vi "Byte Buffer.Read (1D I64).vi"(8 "error in (no error)":errorcluster, 9 "count":i32, 10 "buffer offset":i32, 11 "Byte Buffer in":refnum<class "Byte Buffer.lvclass">) -> (0 "error out":errorcluster, 1 "value":i64[](array[numeric]), 3 "Byte Buffer out":refnum<class "Byte Buffer.lvclass">)   [LabVIEW 2016, in "VeriStand Data.lvlib" / "Byte Buffer.lvclass"]
doc: "Reads <B>count</B> elements of data from the provided <B>Byte Buffer</B> at location <B>buffer offset</B> in the format of the data type specified."
uses:
  Byte Buffer.lvclass
  Byte Buffer.lvclass/Byte Buffer.ctl
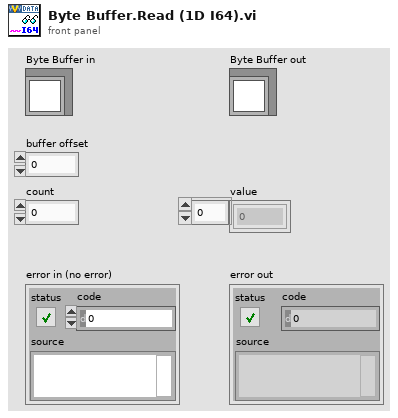
[diagram p1: front panel]
types:
  T1 = enum16{"big-endian, network order", "native, host order", "little-endian"}
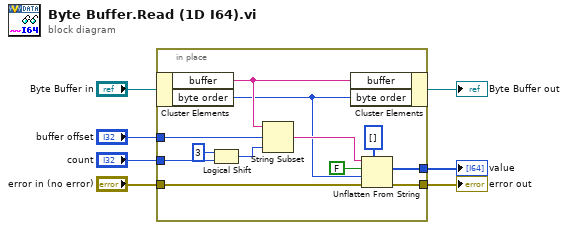
[diagram p0: block diagram]
diagram:
  n1 = in-place {
    in-place-border: "buffer offset" -> [w19]
    in-place-border: "error in (no error)" -> [w17]
    in-place-border: [w14] -> w5
    in-place-border: [w13] -> w4
    in-place-border: "count" -> [w8]
    n2 = in-place-cluster #1("Byte Buffer in") -> ("buffer"=w12:string, "byte order"=w11:T1)
    n3 = Logical Shift(y=i16 3, x=w8) -> (x << y=w9:i32)
    n4 = String Subset(string=w12, offset (0)=w19, length (rest)=w9) -> (substring=w18:string)
    n5 = in-place-cluster #1("buffer"=w12, "byte order"=w11) -> (→"Byte Buffer out":refnum<class "Byte Buffer.lvclass">)
    n6 = Unflatten From String(type=i64[] [], binary string=w18, data includes array or string size? (T)=FALSE, byte order (0:big-endian, network order)=w11, error in (no error)=w17) -> (value=w13:i64[], error out=w14:errorcluster)  [unwired: 1 out]
  }
  "value" <- w4
  "error out" <- w5
